vi "globalSetUp.vi"(8 "error in":errorcluster, 11 "Single Board Loopback in":refnum<class "Octal Loopback.lvclass">) -> (0 "error out":errorcluster, 3 "Single Board Loopback out":refnum<class "Octal Loopback.lvclass">)   [LabVIEW 2020, in "Octal Loopback.lvclass"]
uses:
  Octal Loopback.lvclass
  Octal Loopback.lvclass/Octal Loopback.ctl
  <vilib>/NI/VeriStand Custom Device Testing Tools/VeriStandTestUtilities/VeriStandTestUtilities.lvlib
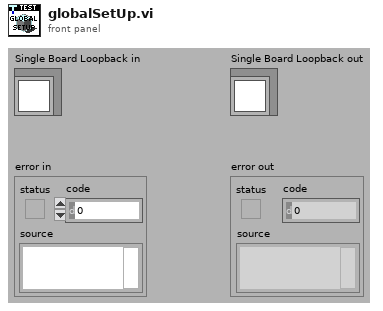
[diagram p1: front panel]
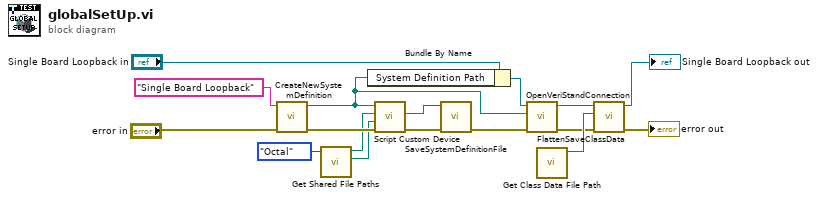
[diagram p0: block diagram]
diagram:
  n1 = call <vilib>:"CreateNewSystemDefinition.vi"("error in"="error in", "System Definition Name"="Single Board Loopback" ("Channel")) -> ("error out"=w14:errorcluster, "System Definition Path"=w5:path)  [unwired: 8 in]
  n2 = call "Get Shared File Paths.vi"("Label Format (Decimal)"=enum16{"Decimal", "Octal"}."Octal") -> ("Hardware File"=w2:path, "Parameters File"=w3:path)  [unwired: 9 in]
  n3 = Bundle By Name(cluster="Single Board Loopback in", "System Definition Path"=w5) -> (w7:refnum<class "Octal Loopback.lvclass">)
  n4 = call "Script Custom Device.vi"("error in"=w14, "Hardware Configuration File Path"=w2, "Parameters Configuration File Path"=w3, "System Definition File Path In"=w5) -> ("error out"=w17:errorcluster, "System Definition Reference"=w12:refnum<k24>)  [unwired: 4 in, 2 out]
  n5 = call <vilib>:"SaveSystemDefinitionFile.vi"("error in (no error)"=w17, "System Definition Reference in"=w12) -> ("error out"=w13:errorcluster)  [unwired: 8 in, 1 out]
  n6 = call-dynamic "OpenVeriStandConnection.vi"("error in (no error)"=w13, "System Definition File"=w5, "VeriStand Test Case in"=w7) -> ("error out"=w8:errorcluster, "VeriStand Test Case out"=w4:refnum<class "Octal Loopback.lvclass">)  [unwired: 6 in, 1 out]
  n7 = call "Get Class Data File Path.vi"() -> ("Class Data File Path"=w9:path)  [unwired: 11 in]
  n8 = call-dynamic "FlattenSaveClassData.vi"("error in"=w8, "Class Data File Path"=w9, "VeriStandTestCase in"=w4) -> ("error out"=→"error out":errorcluster, "VeriStandTestCase out"=→"Single Board Loopback out":refnum<class "Octal Loopback.lvclass">)  [unwired: 7 in]
